vi "파일전송실험.vi"() -> ()   [LabVIEW 2018]
uses:
  <userlib>/_OpenG.lib/largefile/largefile.llb/LF Read File (STR)__ogtk.vi
  <userlib>/_OpenG.lib/largefile/largefile.llb/LF Write File (STR)__ogtk.vi
  <vilib>/Utility/Data Type/NI_Data Type.lvlib
panel:
  in  "Write File":path
  in  "Read File":path
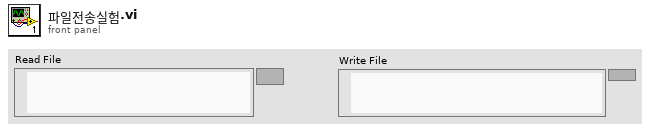
[diagram p1: front panel]
types:
  T1 = enum16{"open", "replace", "create", "open or create", "replace or create", "replace or create with confirmation"}
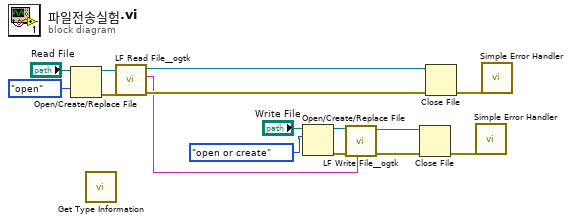
[diagram p0: block diagram]
diagram:
  n1 = Open/Create/Replace File(file path (use dialog)="Read File", operation (0:open)=T1."open" ("동작(0:open)")) -> (refnum out=w8:refnum<file>, error out=w9:errorcluster)  [unwired: 4 in, 1 out]
  n2 = call <vilib>:"Get Type Information.vi"() -> ()  [unwired: 7 in, 5 out]
  n3 = call-poly <userlib>:"LF Read File__ogtk.vi"("error in (no error)"=w9, "refnum"=w8) -> ("error out"=w15:errorcluster, "String"=w11:string, "refnum out"=w14:refnum<file>)  [unwired: 6 in, 1 out]
  n4 = Open/Create/Replace File(file path (use dialog)="Write File", operation (0:open)=T1."open or create" ("동작(0:open)")) -> (refnum out=w6:refnum<file>, error out=w4:errorcluster)  [unwired: 4 in, 1 out]
  n5 = call-poly <userlib>:"LF Write File__ogtk.vi"("data"=w11, "error in (no error)"=w4, "refnum"=w6) -> ("error out"=w13:errorcluster, "refnum out"=w12:refnum<file>)  [unwired: 5 in, 1 out]
  n6 = Close File(refnum=w12, error in=w13) -> (error out=w1:errorcluster)  [unwired: 1 out]
  n7 = Close File(refnum=w14, error in=w15) -> (error out=w2:errorcluster)  [unwired: 1 out]
  n8 = call <vilib>:"Simple Error Handler.vi"("error in (no error)"=w1) -> ()  [unwired: 4 in, 5 out]
  n9 = call <vilib>:"Simple Error Handler.vi"("error in (no error)"=w2) -> ()  [unwired: 4 in, 5 out]
